vi "edit save as.vi"(2 "genneral info":string, 3 "tpdata":string[](array[string]), 4 "appended path":path, 5 "Slide引用句柄":refnum<vi>, 6 "filename":refnum<vi>, 7 "Bool引用句柄":refnum<vi>) -> ()   [LabVIEW 2018]
panel:
  out "genneral info 2":string
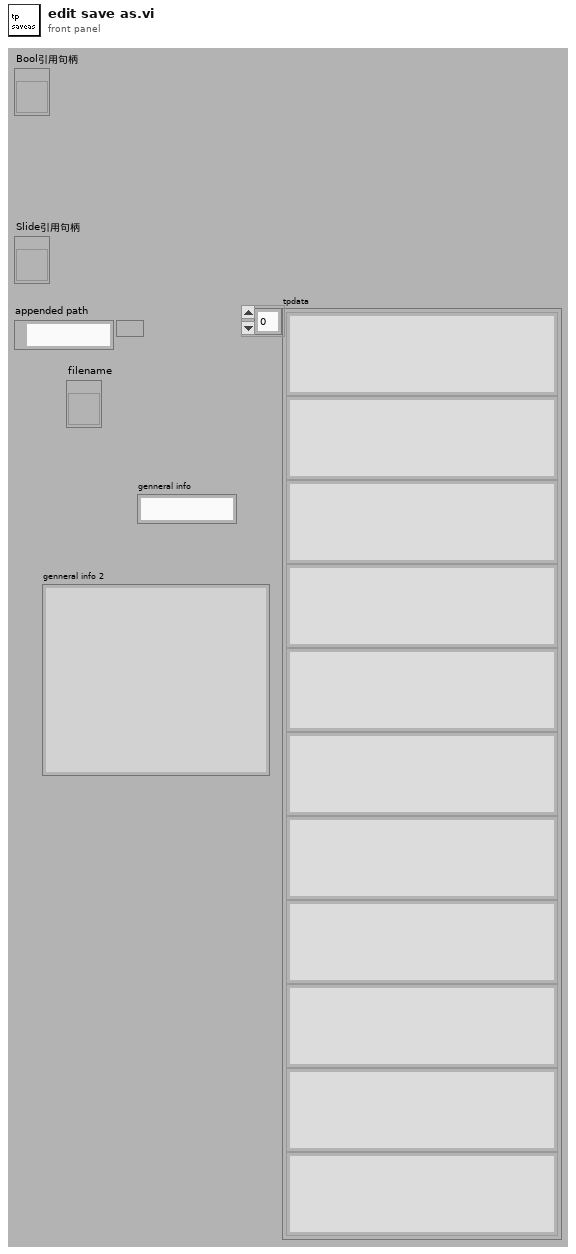
[diagram p1: front panel]
types:
  T1 = enum16{"open", "replace", "create", "open or create", "replace or create", "replace or create with confirmation"}
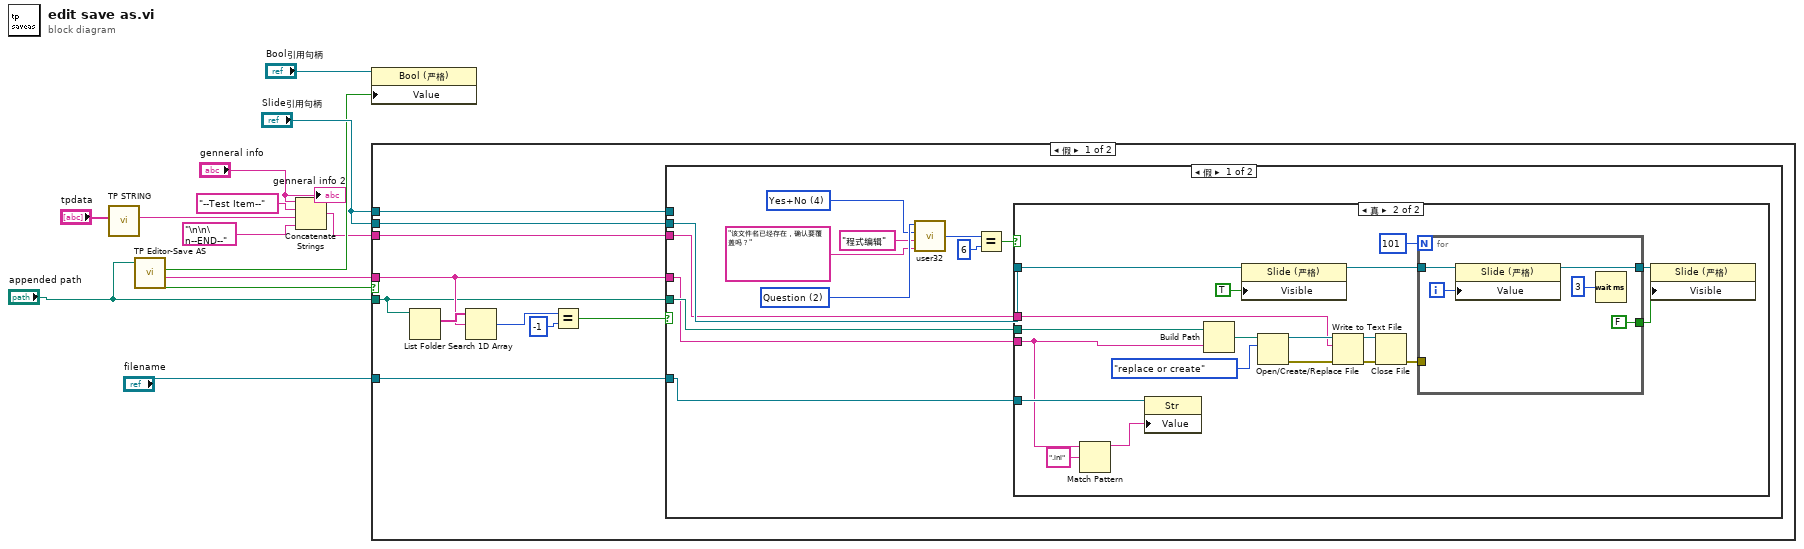
[diagram p0: block diagram]
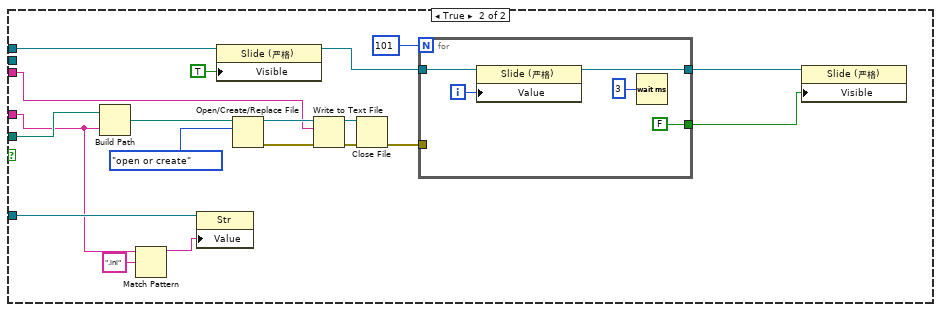
[diagram p3: hidden frame]
diagram:
  n1 = call "TP STRING.vi"("tpdata"="tpdata") -> ("TP OUT"=w7:string)  [unwired: 1 in, 9 out]
  n2 = call "TP Editor-Save AS.vi"("Program path"="appended path") -> (".not. x?"=w11:bool, "Cancel"=w9:bool, "File Name 2"=w10:string)  [unwired: 2 in, 5 out]
  n3 = Concatenate Strings("genneral info", "--Test Item--" ("字符串"), w7, "\n\n\n--END--") -> (w5:string)
  n4 = property on="属性节点" class="Bool (严格)"(reference="Bool引用句柄", "Value"=w11) -> ()  [unwired: 1 in, 2 out]
  n5 = case shown="假" w9 {
    tunnel: "appended path" -> [w18 _]
    tunnel: w10 -> [w19 _]
    tunnel: "Slide引用句柄" -> [w17 _]
    tunnel: "Slide引用句柄" -> [w16 _]
    tunnel: w5 -> [w15 _]
    tunnel: "filename" -> [w14 _]
    frame False {
      n6 = List Folder(path=w18) -> (filenames=w23:string[])  [unwired: 1 in, 5 out]
      n7 = Search 1D Array(1D array=w23, element=w19) -> (index of element=w22:i32)  [unwired: 1 out]
      n8 = Equal?(x=w22, y=-1) -> (x = y?=w20:bool)
      n9 = case shown="假" w20 {
        tunnel: w18 -> [w28 w78]
        tunnel: w19 -> [w27 w61]
        tunnel: w17 -> [w26 _]
        tunnel: w16 -> [_ w69]
        tunnel: w15 -> [w25 w68]
        tunnel: w14 -> [w24 w63]
        frame False {
          w34 = u16 4 items=["OK", "OK+Cancel", "Abort+Retry+Ignore", "Yes+ON+Cancel", "Yes+No", "Retry+Cancel", "Cancel+Retry+Continue"] ("Buttons")
          w35 = u16 2 items=["None", "Critical", "Question", "Exclamation", "Infomation"] ("Icon")
          n10 = call "user32.vi"("Icon"=w35, "Buttons"=w34, "Ipcaption"="程式编辑", "IP Text"="该文件名已经存在，确认要覆盖吗？") -> ("buttin pressed"=w31:i32)  [unwired: 1 out]
          n11 = Equal?(x=w31, y=6) -> (x = y?=w29:bool)
          n12 = case shown="真" w29 {
            tunnel: w28 -> [_ w54]
            tunnel: w27 -> [_ w37]
            tunnel: w26 -> [_ w44]
            tunnel: w25 -> [_ w41]
            tunnel: w24 -> [_ w39]
            frame False {
            }
            frame True {
              n13 = Match Pattern(string=w37, regular expression=".ini" ("正则表达式")) -> (before substring=w36:string)  [unwired: 1 in, 3 out]
              n14 = property on="属性节点" class="Str"(reference=w39, "Value"=w36) -> ()  [unwired: 1 in, 2 out]
              n15 = Build Path(base path=w54, name or relative path=w37) -> (appended path=w53:path)
              n16 = property on="属性节点" class="Slide (严格)"(reference=w44, "Visible"=TRUE) -> (reference out=w43:refnum<vi>)  [unwired: 1 in, 1 out]
              n17 = Open/Create/Replace File(file path (use dialog)=w53, operation (0:open)=T1."replace or create") -> (refnum out=w51:refnum<file>, error out=w50:errorcluster)  [unwired: 1 in, 4 out]
              n18 = Write to Text File(file (use dialog)=w51, text=w41, error in=w50) -> (refnum out=w45:refnum<file>, error out=w46:errorcluster)  [unwired: 2 out]
              n19 = Close File(refnum=w45, error in=w46) -> (error out=w40:errorcluster)  [unwired: 1 out]
              n20 = for {
                N: 101 -> [_]
                tunnel: [FALSE] -> w48
                tunnel: w43 -> [w56]
                tunnel: [w55] -> w42
                tunnel: w40 -> [_]
                i -> [w59]
                n21 = property on="属性节点" class="Slide (严格)"(reference=w56, "Value"=w59) -> (reference out=w55:refnum<vi>)  [unwired: 1 in, 1 out]
                n22 = Wait (ms)(milliseconds to wait=u32 3) -> ()  [unwired: 1 out]
              }
              n23 = property on="属性节点" class="Slide (严格)"(reference=w42, "Visible"=w48) -> ()  [unwired: 1 in, 2 out]
            }
          }
        }
        frame True {
          n24 = Build Path(base path=w78, name or relative path=w61) -> (appended path=w65:path)
          n25 = Match Pattern(string=w61, regular expression=".ini" ("正则表达式")) -> (before substring=w60:string)  [unwired: 1 in, 3 out]
          n26 = property on="属性节点" class="Str"(reference=w63, "Value"=w60) -> ()  [unwired: 1 in, 2 out]
          n27 = property on="属性节点" class="Slide (严格)"(reference=w69, "Visible"=TRUE) -> (reference out=w67:refnum<vi>)  [unwired: 1 in, 1 out]
          n28 = Open/Create/Replace File(file path (use dialog)=w65, operation (0:open)=T1."open or create") -> (refnum out=w76:refnum<file>, error out=w75:errorcluster)  [unwired: 1 in, 4 out]
          n29 = Write to Text File(file (use dialog)=w76, text=w68, error in=w75) -> (refnum out=w74:refnum<file>, error out=w71:errorcluster)  [unwired: 2 out]
          n30 = Close File(refnum=w74, error in=w71) -> (error out=w64:errorcluster)  [unwired: 1 out]
          n31 = for {
            N: 101 -> [_]
            tunnel: [FALSE] -> w72
            tunnel: w67 -> [w80]
            tunnel: [w79] -> w66
            tunnel: w64 -> [_]
            i -> [w83]
            n32 = property on="属性节点" class="Slide (严格)"(reference=w80, "Value"=w83) -> (reference out=w79:refnum<vi>)  [unwired: 1 in, 1 out]
            n33 = Wait (ms)(milliseconds to wait=u32 3) -> ()  [unwired: 1 out]
          }
          n34 = property on="属性节点" class="Slide (严格)"(reference=w66, "Visible"=w72) -> ()  [unwired: 1 in, 2 out]
        }
      }
    }
    frame True {
    }
  }
  "genneral info 2" <- "genneral info"
